vi "FTW-STR-Display-Bytes.vi"(0 "Bytes":i64, 1 "Display Style":T1(ring)) -> (2 "Display":string)   [LabVIEW 2012]
panel:
  # "Inputs"
  # "Outputs"
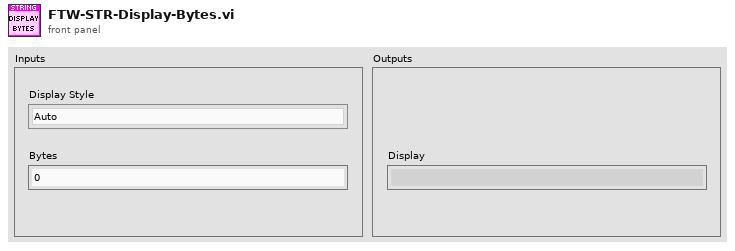
[diagram p1: front panel]
types:
  T1 = enum16{"Auto", "Plain Bytes", "000 bytes", "0.00kB", "0.00MB", "0.00GB", "0.00TB"}
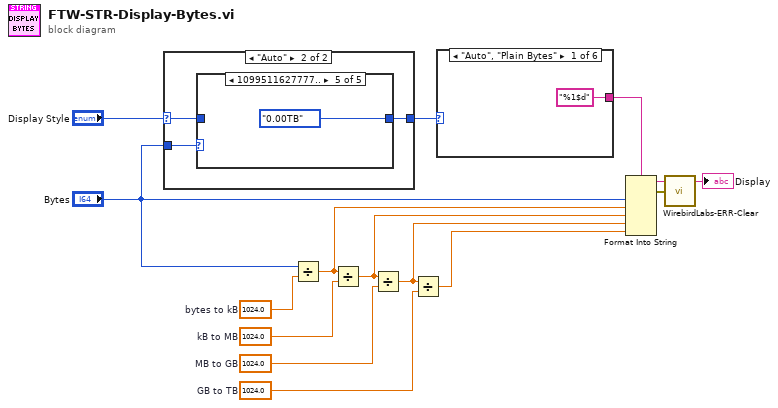
[diagram p0: block diagram]
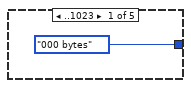
[diagram p3: hidden frame]
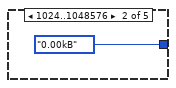
[diagram p4: hidden frame]
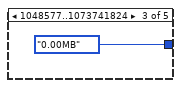
[diagram p5: hidden frame]
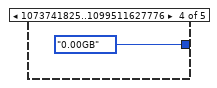
[diagram p6: hidden frame]
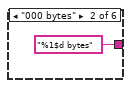
[diagram p7: hidden frame]
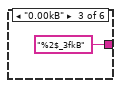
[diagram p8: hidden frame]
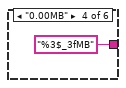
[diagram p9: hidden frame]
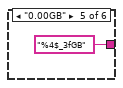
[diagram p10: hidden frame]
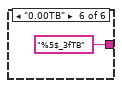
[diagram p11: hidden frame]
diagram:
  w9 = 1024.0  # GB to TB
  w10 = 1024.0  # MB to GB
  w11 = 1024.0  # kB to MB
  w12 = 1024.0  # bytes to kB
  n1 = case shown="\"Auto\"" "Display Style" {
    selector: "Display Style" -> [w15 w17]
    tunnel: "Bytes" -> [_ w18]
    tunnel: [w15 w16] -> w1
    frame Default {
    }
    frame "Auto" {
      n2 = case shown="1099511627777.." w18 {
        tunnel: w17 -> [_ _ _ _ _]
        tunnel: [T1."000 bytes" ("Display Style") T1."0.00kB" ("Display Style") T1."0.00MB" ("Display Style") T1."0.00GB" ("Display Style") T1."0.00TB" ("Display Style")] -> w16
        frame ..1023 {
        }
        frame 1024..1048576 {
        }
        frame 1048577..1073741824 {
        }
        frame 1073741825..1099511627776 {
        }
        frame 1099511627777.. {
        }
      }
    }
  }
  n3 = Divide(x="Bytes", y=w12) -> (x/y=w8:dbl)
  n4 = Divide(x=w8, y=w11) -> (x/y=w7:dbl)
  n5 = Divide(x=w7, y=w10) -> (x/y=w6:dbl)
  n6 = Divide(x=w6, y=w9) -> (x/y=w5:dbl)
  n7 = case shown="\"Auto\", \"Plain Bytes\"" w1 {
    tunnel: ["%1$d" "%1$d bytes" "%2$_3fkB" "%3$_3fMB" "%4$_3fGB" "%5$_3fTB"] -> w14
    frame "Auto", "Plain Bytes" {
    }
    frame "000 bytes" {
    }
    frame "0.00kB" {
    }
    frame "0.00MB" {
    }
    frame "0.00GB" {
    }
    frame "0.00TB" {
    }
  }
  n8 = Format Into String(format string=w14, "Bytes", w8, w7, w6, w5) -> (resulting string=→"Display":string, error out=w13:errorcluster)  [unwired: 2 in]
  n9 = call "WirebirdLabs-ERR-Clear.vi"("error to snuff"=w13) -> ()  [unwired: 1 out]
